vi "Save to file.vi"(8 "error in (no error)":errorcluster, 11 "Loop Data":T1) -> (0 "error out":errorcluster)   [LabVIEW 2015]
uses:
  TypDefs/Loop Data.ctl
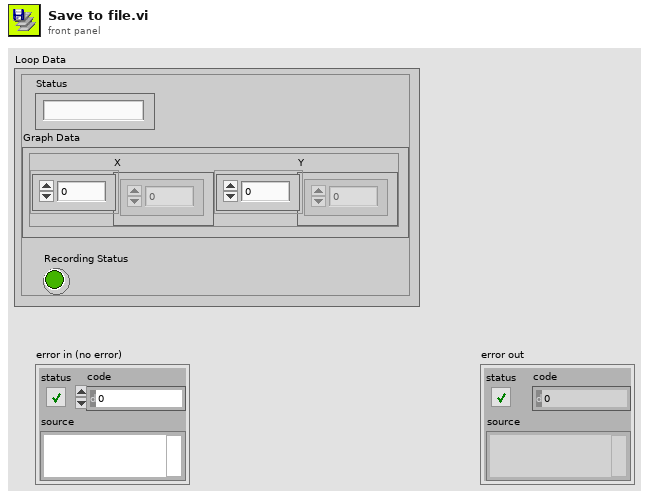
[diagram p1: front panel]
types:
  T1 = typedef "Loop Data.ctl" = cluster{"Status":string, "Graph Data":cluster{"X":dbl[], "Y":dbl[]}, "Recording Status":bool}
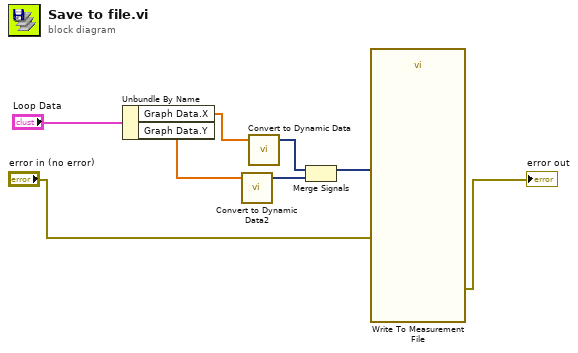
[diagram p0: block diagram]
diagram:
  n1 = Unbundle By Name("Loop Data") -> ("Graph Data.X"=w7:dbl[], "Graph Data.Y"=w4:dbl[])
  n2 = call "Convert to Dynamic Data2"("Array"=w4) -> ("Dynamic Data Type"=w3:dynamicdata)  [unwired: 3 in]
  n3 = call "Convert to Dynamic Data"("Array"=w7) -> ("Dynamic Data Type"=w6:dynamicdata)  [unwired: 3 in]
  n4 = Merge Signals(w6, w3) -> (w5:dynamicdata)
  n5 = call "Write To Measurement File"("Signals"=w5, "error in (no error)"="error in (no error)") -> ("error out"=→"error out":errorcluster)  [unwired: 15 in, 2 out]
